vi "SLT2MTStepName.vi"(10 "StationIn":string) -> (2 "StationOut":string)   [LabVIEW 2012]
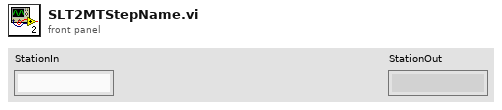
[diagram p1: front panel]
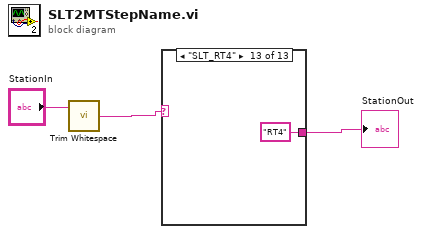
[diagram p0: block diagram]
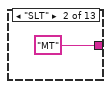
[diagram p3: hidden frame]
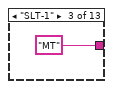
[diagram p4: hidden frame]
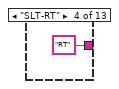
[diagram p5: hidden frame]
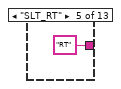
[diagram p6: hidden frame]
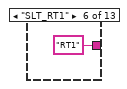
[diagram p7: hidden frame]
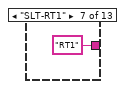
[diagram p8: hidden frame]
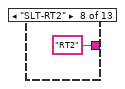
[diagram p9: hidden frame]
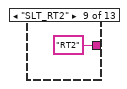
[diagram p10: hidden frame]
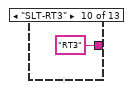
[diagram p11: hidden frame]
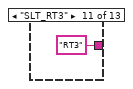
[diagram p12: hidden frame]
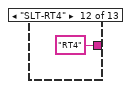
[diagram p13: hidden frame]
diagram:
  n1 = call <vilib>:"Trim Whitespace.vi"("string"="StationIn") -> ("trimmed string"=w2:string)  [unwired: 1 in]
  n2 = case shown="\"SLT_RT4\"" w2 {
    selector: w2 -> [w4 _ _ _ _ _ _ _ _ _ _ _ _]
    tunnel: [w4 "MT" "MT" "RT" "RT" "RT1" "RT1" "RT2" "RT2" "RT3" "RT3" "RT4" "RT4"] -> w1
    frame "False", Default {
    }
    frame "SLT" {
    }
    frame "SLT-1" {
    }
    frame "SLT-RT" {
    }
    frame "SLT_RT" {
    }
    frame "SLT_RT1" {
    }
    frame "SLT-RT1" {
    }
    frame "SLT-RT2" {
    }
    frame "SLT_RT2" {
    }
    frame "SLT-RT3" {
    }
    frame "SLT_RT3" {
    }
    frame "SLT-RT4" {
    }
    frame "SLT_RT4" {
    }
  }
  "StationOut" <- w1
